vi "Pokayoke_Check.vi"(6 "Tag Name":string, 7 "Pokayoke Data":variant[][](array[variant]), 8 "RFID":string, 10 "Table":string, 11 "Ref in":T1={"MS SQL Connection"=refnum, "UDL File"=path "", "Time"="", "DCODE"="", "WIP+1"=0, "MC No?"=0, "POKAYOKE?"=FALSE, "Expected Result"="", "Result [Status]"="", "Clock"=0.0, "RFID"="", "WIP Queue"=refnum, "TS Parameter"={"ProfitCenterCode"="", "LineCode"="", "WorkOrderNumber"="", "Model"="", "Model_with_Prefix"="", "VendorCode"="", "SetParameterDateCode"="", "PokaYoke"=0, "Target"=1, "Live_DateCode"="", "CustomerPartNumber"="", "Hand"="", "sBarcode"=FALSE, "FCA"=0, "Ent_Stamp"=timestamp(0 s since 1904-01-01), "STS_CD"=0.0}, "Data_Queue"=[], "RFID Serial No."=""} {"TS Parameter"."FCA" format="%01d"; "TS Parameter"."Target" min=1 max=100000; "TS Parameter"."PokaYoke" min=0 max=1}) -> (1 "TS_BSC":i32, 2 "TS_Message":string, 4 "Message":picture, 5 "Expected Result":string)   [LabVIEW 2020]
uses:
  Controls/TD SQL.ctl
  <vilib>/addons/database/Connection.llb/Conn ObjectReference.ctl
  Controls/WIP_State.ctl
  Controls/TS_Parameter.ctl
  Controls/Msg_Type.ctl
  Controls/Status.ctl
  MS SQL/MS_Global.vi
  <vilib>/addons/database/NI_Database_API.lvlib
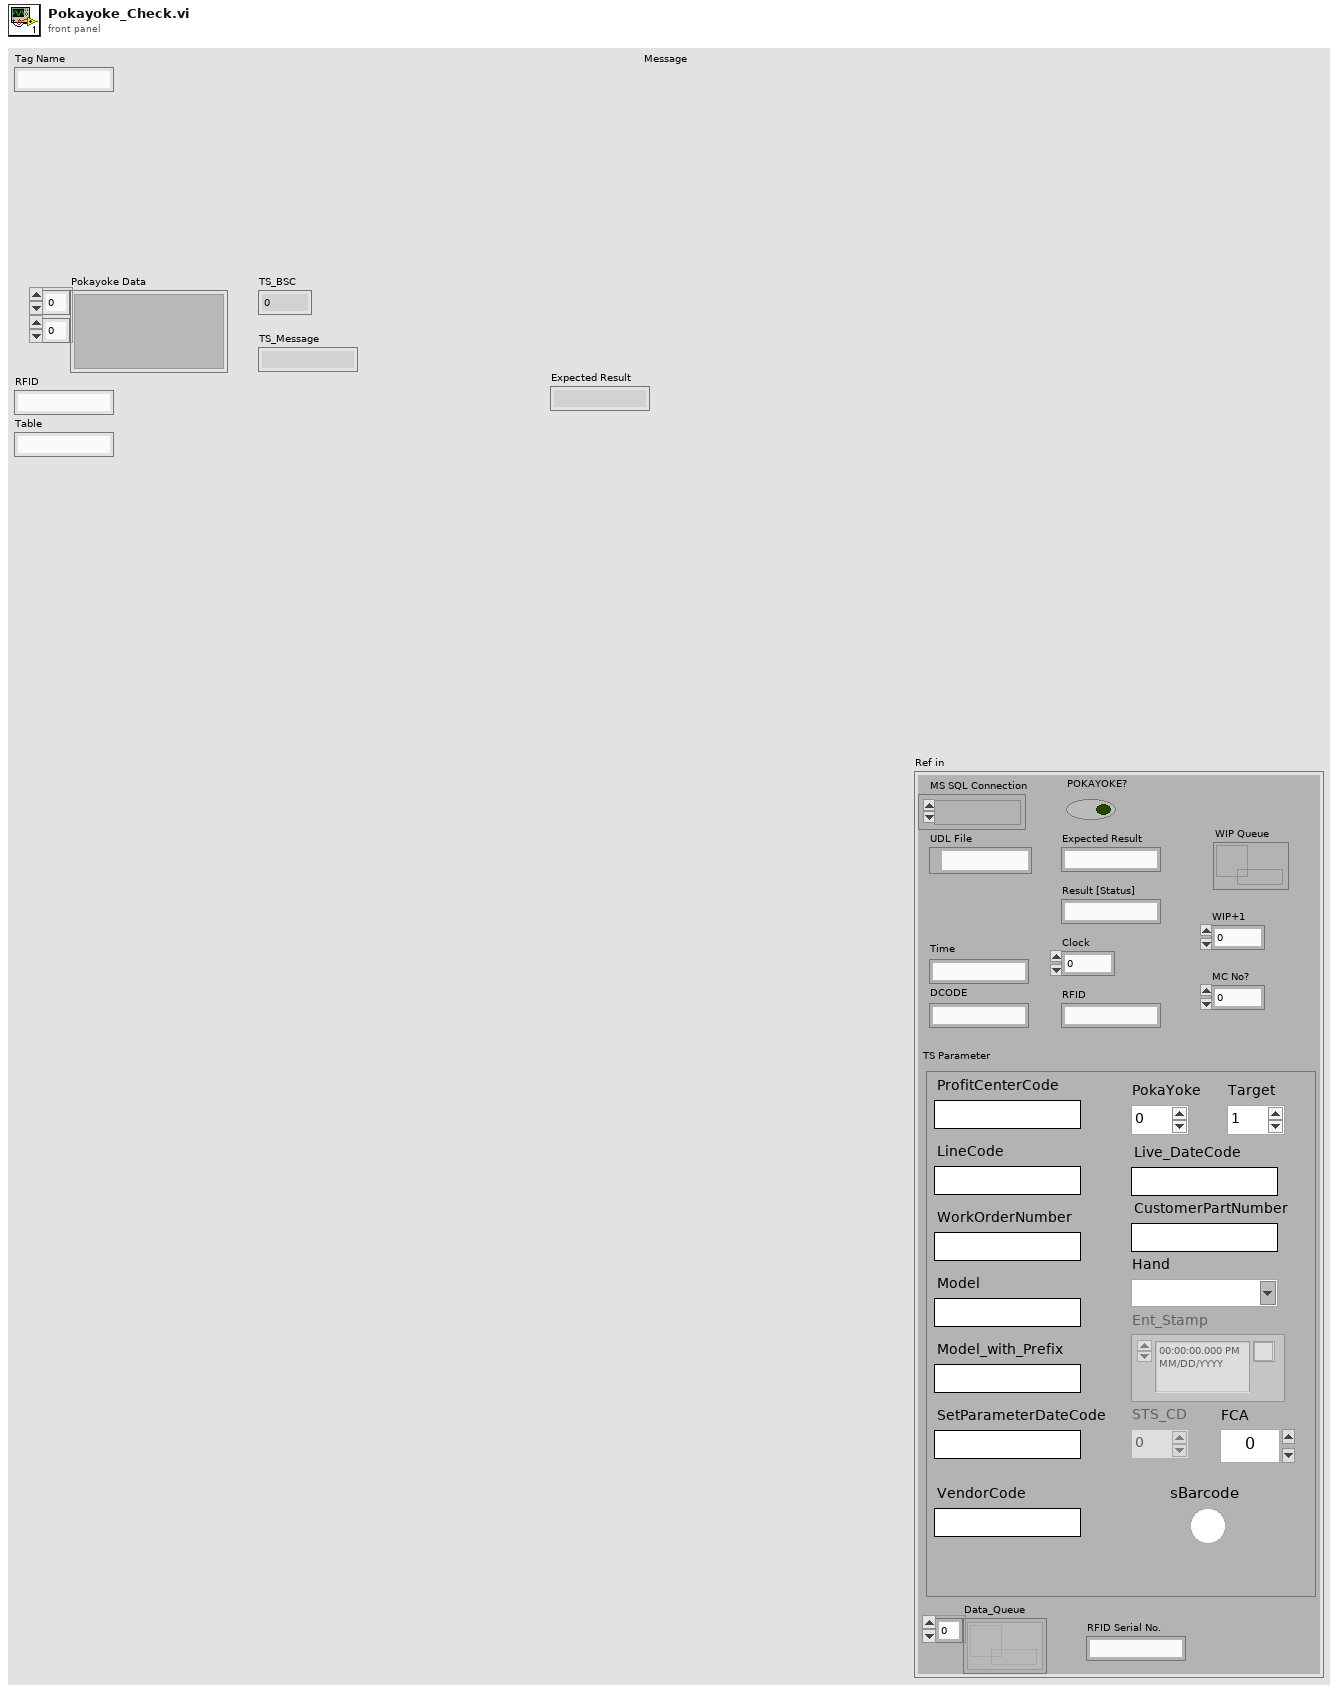
[diagram p1: front panel]
types:
  T1 = typedef "TD SQL.ctl" = cluster{"MS SQL Connection":T2, "UDL File":path, "Time":string, "DCODE":string, "WIP+1":i64, "MC No?":i32, "POKAYOKE?":bool, "Expected Result":string, "Result [Status]":string, "Clock":dbl, "RFID":string, "WIP Queue":refnum<queue>, "TS Parameter":T3, "Data_Queue":refnum<queue>[], "RFID Serial No.":string}
  T2 = typedef "NI_Database_API.lvlib/Conn ObjectReference.ctl" = refnum<k1>
  T3 = typedef "TS_Parameter.ctl" = cluster{"ProfitCenterCode":string, "LineCode":string, "WorkOrderNumber":string, "Model":string, "Model_with_Prefix":string, "VendorCode":string, "SetParameterDateCode":string, "PokaYoke":i32, "Target":i32, "Live_DateCode":string, "CustomerPartNumber":string, "Hand":string, "sBarcode":bool, "FCA":i32, "Ent_Stamp":timestamp, "STS_CD":dbl}
  T4 = typedef "Msg_Type.ctl" = enum16{"Normal", "Pass", "Fail", "Fault", "User", "Bypass", "Fail Save"}
  T5 = typedef "Status.ctl" = u16
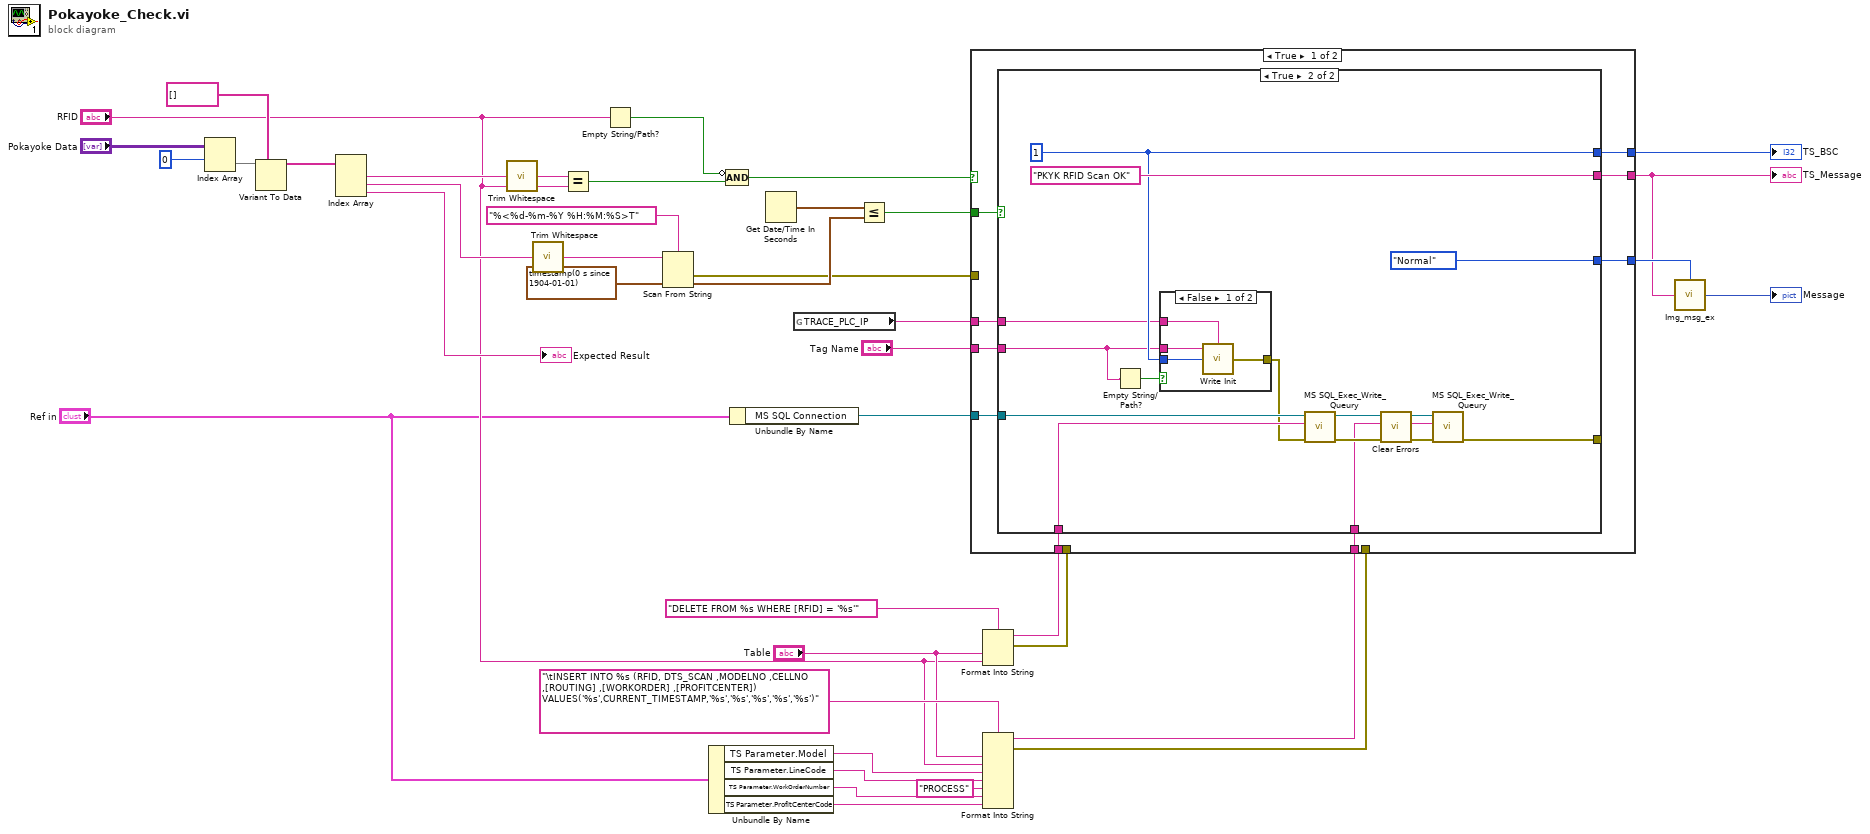
[diagram p0: block diagram]
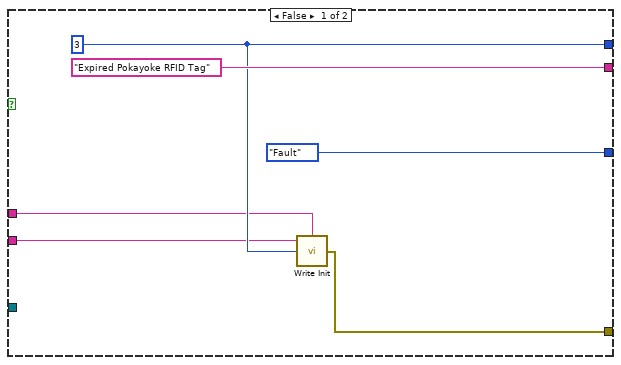
[diagram p2: hidden frame]
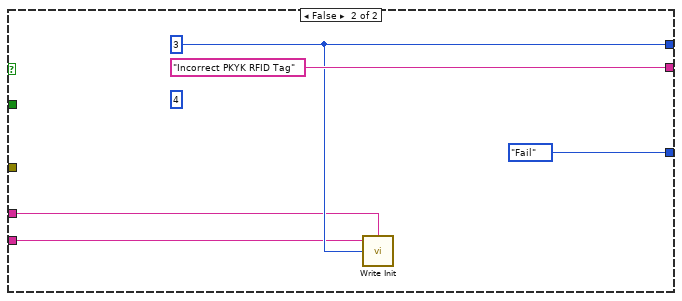
[diagram p4: hidden frame]
diagram:
  n1 = Index Array(array="Pokayoke Data", index (row)=0) -> (element=w37:variant[])  [unwired: 1 in]
  n2 = Variant To Data(type=string[] [], Variant=w37) -> (data=w35:string[])  [unwired: 1 in, 1 out]
  n3 = Index Array(array=w35) -> (element #1=w34:string, element #2=w29:string, element #3=→"Expected Result":string)  [unwired: 3 in]
  n4 = call <vilib>:"Trim Whitespace.vi"("string"=w34) -> ("trimmed string"=w33:string)  [unwired: 1 in]
  n5 = call <vilib>:"Trim Whitespace.vi"("string"=w29) -> ("trimmed string"=w28:string)  [unwired: 1 in]
  n6 = Equal?(x=w33, y="RFID") -> (x = y?=w32:bool)
  n7 = Empty String/Path?(string/path="RFID") -> (empty?=w22:bool)
  n8 = Scan From String(format string="%<%d-%m-%Y %H:%M:%S>T" ("time format string (%c)"), input string=w28, default 1=timestamp(0 s since 1904-01-01) ("time stamp")) -> (error out=w21:errorcluster, output 1=w25:timestamp)  [unwired: 2 in, 2 out]
  n9 = Unbundle By Name("Ref in") -> ("TS Parameter.Model"=w4:string, "TS Parameter.LineCode"=w3:string, "TS Parameter.WorkOrderNumber"=w2:string, "TS Parameter.ProfitCenterCode"=w1:string)
  n10 = Compound Arithmetic op=AND(invert w22, w32) -> (w23:bool)
  n11 = Unbundle By Name("Ref in") -> ("MS SQL Connection"=w19:T2)
  n12 = Get Date/Time In Seconds() -> (seconds since 1Jan1904=w26:timestamp)
  n13 = global read "MS_Global.vi" "TRACE_PLC_IP"() -> (w6:string)
  n14 = Less Or Equal?(x=w26, y=w25) -> (x <= y?=w24:bool)
  n15 = Format Into String(format string="DELETE FROM %s WHERE [RFID] = '%s'" ("Query"), "Table", "RFID") -> (resulting string=w18:string, error out=w17:errorcluster)  [unwired: 2 in]
  n16 = Format Into String(format string="\tINSERT INTO %s (RFID, DTS_SCAN ,MODELNO ,CELLNO ,[ROUTING] ,[WORKORDER] ,[PROFITCENTER]) VALUES('%s',CURRENT_TIMESTAMP,'%s','%s','%s','%s','%s')", "Table", "RFID", w4, w3, "PROCESS" ("input 5"), w2, w1) -> (resulting string=w12:string, error out=w13:errorcluster)  [unwired: 2 in]
  n17 = case shown="True" w23 {
    tunnel: [w49 w76] -> w40
    tunnel: [w48 "Incorrect PKYK RFID Tag"] -> w8
    tunnel: w24 -> [w47 _]
    tunnel: w21 -> [_ _]
    tunnel: w19 -> [w46 _]
    tunnel: w18 -> [w45 _]
    tunnel: w17 -> [_ _]
    tunnel: w13 -> [_ _]
    tunnel: w12 -> [w44 _]
    tunnel: "Tag Name" -> [w43 w75]
    tunnel: [w42 Msg_Type."Fail" ("Msg Type")] -> w9
    tunnel: w6 -> [w41 w74]
    frame True {
      n18 = case shown="True" w47 {
        tunnel: [w53 w60] -> w49
        tunnel: ["Expired Pokayoke RFID Tag" "PKYK RFID Scan OK"] -> w48
        tunnel: w46 -> [_ w68]
        tunnel: w45 -> [_ w67]
        tunnel: w44 -> [_ w64]
        tunnel: [w51 w62] -> _
        tunnel: w43 -> [w52 w58]
        tunnel: [Msg_Type."Fault" ("Msg Type") Msg_Type."Normal" ("Msg Type")] -> w42
        tunnel: w41 -> [w50 w56]
        frame False {
          w53 = 3 ("TS_BSC")
          n19 = call "Write Init.vi"("Network Path"=w50, "Int"=w53, "Tag Name"=w52) -> ("error out"=w51:errorcluster)  [unwired: 1 in]
        }
        frame True {
          w60 = 1 ("TS_BSC")
          n20 = Empty String/Path?(string/path=w58) -> (empty?=w61:bool)
          n21 = case shown="False" w61 {
            tunnel: w56 -> [w73 _]
            tunnel: w60 -> [w72 _]
            tunnel: [w71 _] -> w59
            tunnel: w58 -> [w70 _]
            frame False {
              n22 = call "Write Init.vi"("Network Path"=w73, "Int"=w72, "Tag Name"=w70) -> ("error out"=w71:errorcluster)  [unwired: 1 in]
            }
            frame True {
            }
          }
          n23 = call "MS SQL_Exec_Write_Queury.vi"("error in (no error)"=w59, "Query"=w67, "Refnum in"=w68) -> ("error out"=w65:errorcluster, "Refnum out"=w66:T2)  [unwired: 7 in]
          n24 = call <vilib>:"Clear Errors.vi"("error in (no error)"=w65) -> ("error out"=w63:errorcluster)  [unwired: 5 in, 1 out]
          n25 = call "MS SQL_Exec_Write_Queury.vi"("error in (no error)"=w63, "Query"=w64, "Refnum in"=w66) -> ("error out"=w62:errorcluster)  [unwired: 7 in, 1 out]
        }
      }
    }
    frame False {
      (unwired) T5 4 ("pStatus")
      w76 = 3 ("TS_BSC")
      n26 = call "Write Init.vi"("Network Path"=w74, "Int"=w76, "Tag Name"=w75) -> ()  [unwired: 1 in, 1 out]
    }
  }
  "TS_BSC" <- w40
  "TS_Message" <- w8
  n27 = call "Img_msg_ex.vi"("Msg Type"=w9, "Message In"=w8) -> ("Message"=→"Message":picture)  [unwired: 2 in]
